vi "Configure Modulation (PSK).vi"(5 "Channel (1:Channel 1)":i32(ring)=1 items=["Channel 1"=1, "Channel 2"=2], 6 "Key Frequency (100.000 Hz)":dbl=100.0 format="%.3f", 7 "Enable PSK Modulation (T:Enable)":bool=TRUE, 8 "error in (no error)":errorcluster, 9 "Polarity (0: Positive)":u16(ring) items=["Positive", "Negative"], 10 "PSK Source (0: Internal)":u16(ring) items=["Internal", "External"], 11 "VISA resource name":refnum<visa-resource-name>) -> (0 "error out":errorcluster, 3 "VISA resource name out":refnum<visa-resource-name>)   [LabVIEW 2015, in "SDG X Series.lvlib"]
doc: "Configures and enables PSK modulation for the SDG2000X/E series.\n\n<B>Note:</B> The carrier waveform shape and parameters are set by the Configure Standard Waveform VI."
uses:
  <instrlib>/SDG X Series/SDG X Series.lvlib
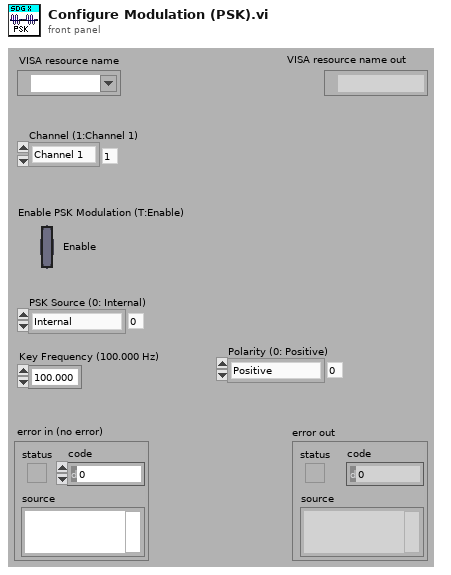
[diagram p1: front panel]
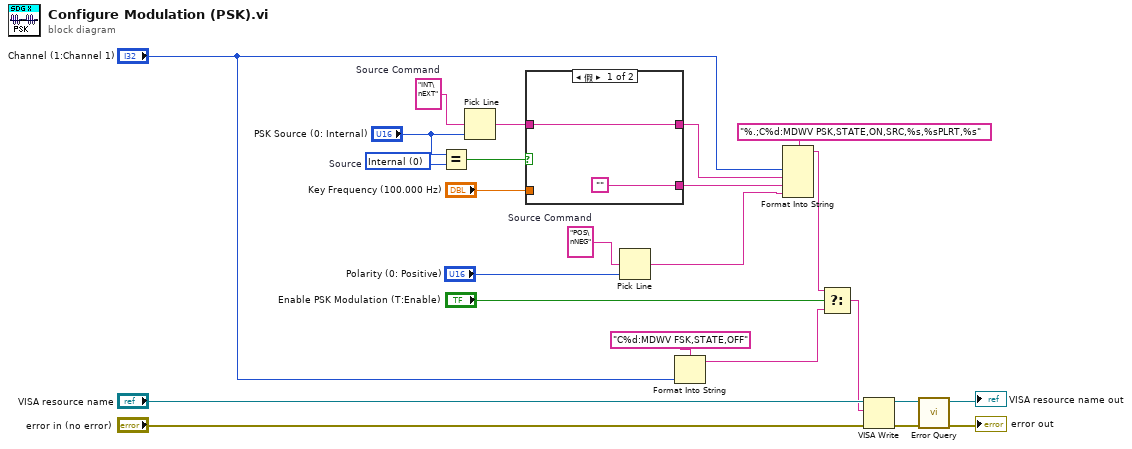
[diagram p0: block diagram]
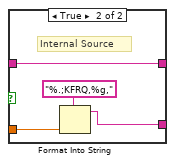
[diagram p2: hidden frame]
diagram:
  w3 = "POS\nNEG"  # Source Command
  w17 = "INT\nEXT"  # Source Command
  w13 = u16 0 items=["Internal", "External"]  # Source
  n1 = Equal?(x="PSK Source (0: Internal)", y=w13) -> (x = y?=w16:bool)
  n2 = Pick Line(multi-line string=w17, line index="PSK Source (0: Internal)") -> (output string=w15:string)  [unwired: 1 in]
  n3 = case shown="假" w16 {
    tunnel: w15 -> [w26 w30]
    tunnel: [w26 w30] -> w11
    tunnel: ["" w27] -> w2
    tunnel: "Key Frequency (100.000 Hz)" -> [_ w28]
    frame False {
    }
    frame True {
      # "Internal Source"
      n4 = Format Into String(format string="%.;KFRQ,%g,", w28) -> (resulting string=w27:string)  [unwired: 2 in, 1 out]
    }
  }
  n5 = Pick Line(multi-line string=w3, line index="Polarity (0: Positive)") -> (output string=w1:string)  [unwired: 1 in]
  n6 = Format Into String(format string="C%d:MDWV FSK,STATE,OFF", "Channel (1:Channel 1)") -> (resulting string=w8:string)  [unwired: 2 in, 1 out]
  n7 = Format Into String(format string="%.;C%d:MDWV PSK,STATE,ON,SRC,%s,%sPLRT,%s", "Channel (1:Channel 1)", w11, w2, w1) -> (resulting string=w7:string)  [unwired: 2 in, 1 out]
  n8 = Select(t=w7, s="Enable PSK Modulation (T:Enable)", f=w8) -> (s? t:f=w6:string)
  n9 = VISA Write(VISA resource name="VISA resource name", write buffer=w6, error in (no error)="error in (no error)") -> (VISA resource name out=w22:refnum<visa-resource-name>, error out=w21:errorcluster)  [unwired: 1 out]
  n10 = call <instrlib>:"Error Query.vi"("error in (no error)"=w21, "VISA resource name"=w22) -> ("error out"=→"error out":errorcluster, "VISA resource name out"=→"VISA resource name out":refnum<visa-resource-name>)  [unwired: 6 in, 2 out]
